vi "KE6221 -- Test Set Get Arb Waveform Points tmp.vi"() -> ()   [LabVIEW 2014, in "Keithley 622x tmp.lvlib"]
uses:
  Keithley 622x tmp.lvlib
  Typedefs/KE6221 -- Wave Arb Point.ctl
  Typedefs/KE6221 -- Arb Location.ctl
panel:
  in  "Arb Location":T1
  out "Delta Sum":T2 min=-1.0 max=1.0 format="%.6g"
  out "Delta":dbl[](graph)
  out "Plot":dbl[][](graph)
  out "error out":errorcluster
  out "Arb Waveform Points Out":T2[](array[typedef]) min=-1.0 max=1.0 format="%.3f"
  out "Num Points Out":u32
  out "Arb Points In":dbl[](array[numeric]) format="%.3f"
  in  "Resource In":refnum<visa-resource-name>
  in  "Min Val":dbl=-1.0 min=-1.0 max=0.0 format="%.3f"
  in  "Max Val":dbl=1.0 min=0.0 max=1.0 format="%.3f"
  in  "Num Points":u32
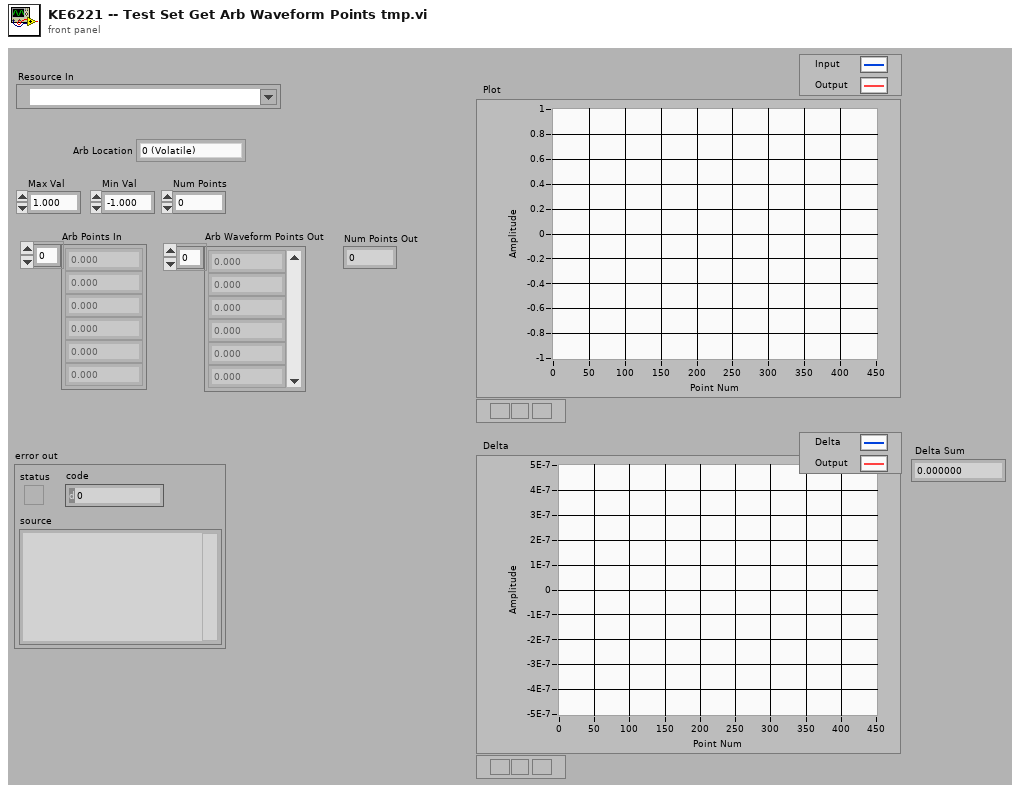
[diagram p1: front panel]
types:
  T1 = typedef "Keithley 622x tmp.lvlib/KE6221 -- Arb Location.ctl" = enum16{"0 (Volatile)", "1 (NVRAM)", "2 (NVRAM)", "3 (NVRAM)", "4 (NVRAM)"}
  T2 = typedef "Keithley 622x tmp.lvlib/KE6221 -- Wave Arb Point.ctl" = dbl
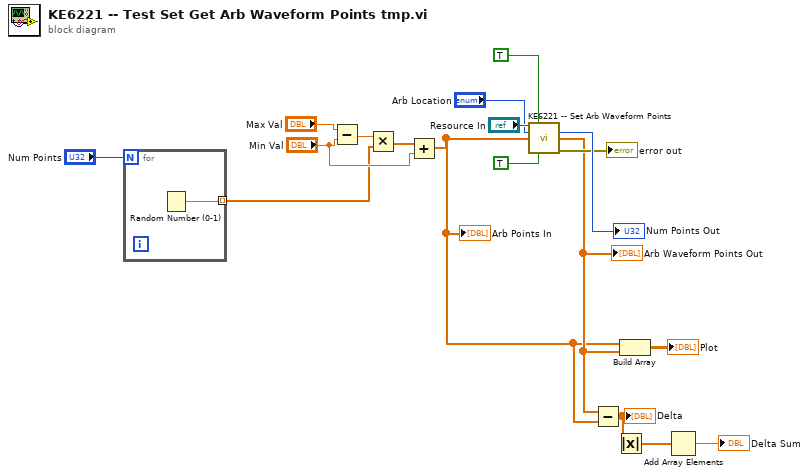
[diagram p0: block diagram]
diagram:
  n1 = for {
    N: "Num Points" -> [_]
    tunnel: [w19] -> w13 mode=indexing
    n2 = Random Number (0-1)() -> (number: 0 to 1=w19:dbl)
  }
  n3 = Subtract(x="Max Val", y="Min Val") -> (x-y=w16:dbl)
  n4 = Multiply(x=w16, y=w13) -> (x*y=w15:dbl[])
  n5 = Add(x=w15, y="Min Val") -> (x+y=w5:dbl[])
  "Arb Points In" <- w5
  n6 = call "KE6221 -- Set Arb Waveform Points.vi"("Resource In"="Resource In", "Check For SCPI Errors? (T)"=TRUE, "Arb Location"="Arb Location", "Arb Waveform Points In"=w5, "Read Back Set Values? (T)"=TRUE ("Read Back Set Value? (T)")) -> ("Num Points Out"=→"Num Points Out":u32, "Arb Waveform Points Out"=w6:T2[], "error out"=→"error out":errorcluster)  [unwired: 7 in, 1 out]
  "Arb Waveform Points Out" <- w6
  n7 = Subtract(x=w6, y=w5) -> (x-y=w4:T2[])
  "Delta" <- w4
  n8 = Absolute Value(x=w4) -> (abs(x)=w2:T2[])
  n9 = Build Array(w5, w6) -> (→"Plot":T2[][])
  n10 = Add Array Elements(numeric array=w2) -> (sum=→"Delta Sum":T2)
